vi "G4SubTemplate_Simple_6x8x6_Create.vi"(0 "reference in":refnum<class "G4SubTemplate_Simple_6x8x6.lvclass">, 5 "Error In":errorcluster) -> (14 "reference out":refnum<class "G4SubTemplate_Simple_6x8x6.lvclass">, 19 "Error Out":errorcluster)   [LabVIEW 2020, in "G4SubTemplate_Simple_6x8x6.lvclass"]
uses:
  G4SubTemplate_Simple_6x8x6.lvclass
  C:/VIT/GitHub/OpenGDS/resource/Framework/Providers/Open_GDS/ClassProviders/Provider_EndevoGOOP400/Templates/G4BaseTemplate_Simple_6x8x6/G4BaseTemplate_Simple_6x8x6.lvclass
  G4BaseTemplate_Simple_6x8x6/G4BaseTemplate_Simple_6x8x6.lvclass
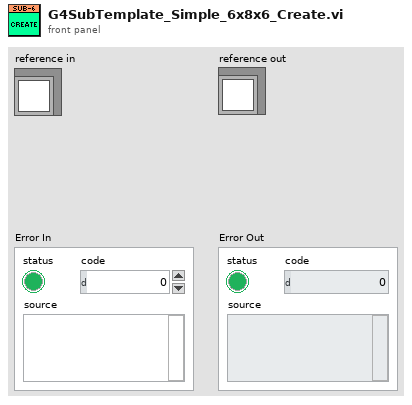
[diagram p1: front panel]
types:
  T1 = typedef "G4SubTemplate_Simple_6x8x6.lvclass/ObjectAttributes.ctl" = cluster{"Attribute1":dbl}
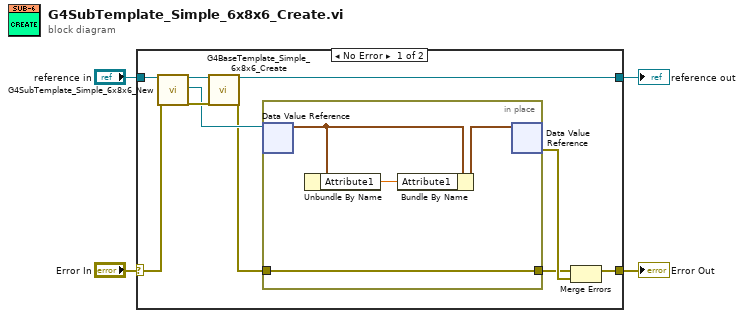
[diagram p0: block diagram]
diagram:
  n1 = case shown="No Error" "Error In" {
    selector: "Error In" -> [w13 w20]
    tunnel: [w11 w20] -> w3
    tunnel: "reference in" -> [w14 w19]
    tunnel: [w8 w19] -> w1
    frame No Error {
      n2 = call "G4SubTemplate_Simple_6x8x6_New.vi"("reference in"=w14, "Error In"=w13) -> ("reference out"=w10:refnum<class "G4SubTemplate_Simple_6x8x6.lvclass">, "DVRRefOut"=w7:refnum<data-value>, "Error Out"=w9:errorcluster)  [unwired: 14 in, 1 out]
      n3 = call "G4BaseTemplate_Simple_6x8x6_Create.vi"("reference in"=w10, "Error In"=w9) -> ("reference out"=w8:refnum<class "G4SubTemplate_Simple_6x8x6.lvclass">, "Error Out"=w6:errorcluster)  [unwired: 16 in]
      n4 = in-place {
        in-place-border: w6 -> [w15]
        in-place-border: [w15] -> w5
        n5 = in-place-dvr #1(w7) -> (w17:T1)  [unwired: 1 out]
        n6 = Unbundle By Name(w17) -> ("Attribute1"=w16:dbl)
        n7 = Bundle By Name(cluster=w17, "Attribute1"=w16) -> (w18:T1)
        n8 = in-place-dvr #1(w18) -> (w12:errorcluster)  [unwired: 1 out]
      }
      n9 = Merge Errors(w5, w12) -> (w11:errorcluster)
    }
    frame Error {
    }
  }
  "Error Out" <- w3
  "reference out" <- w1
